vi "Set_Driver.vi"(8 "error in (no error)":errorcluster caption="错误输入（无错误）", 10 "Driver":string[](array[string]), 11 "文件路径 ：":path) -> (0 "error out":errorcluster, 3 "dup path":path)   [LabVIEW 2018]
uses:
  <vilib>/Utility/config.llb/Write Key (String).vi
  <vilib>/Utility/config.llb/NI_LVConfig.lvlib
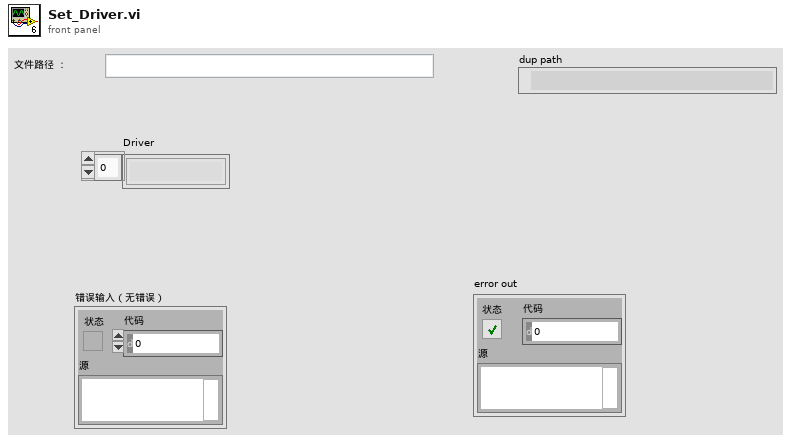
[diagram p1: front panel]
types:
  T1 = enum16{"open", "replace", "create", "open or create", "replace or create", "replace or create with confirmation"}
  T2 = typedef "NI_LVConfig.lvlib/Config Data RefNum.ctl" = refnum<k1>
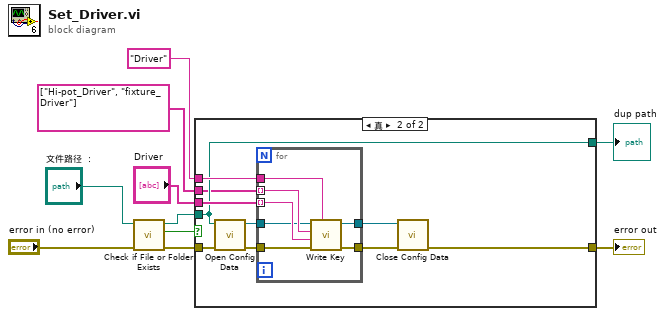
[diagram p0: block diagram]
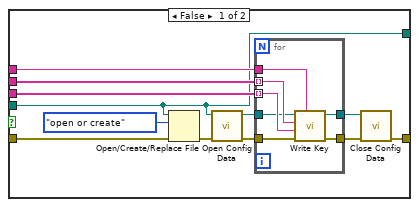
[diagram p2: hidden frame]
diagram:
  n1 = call <vilib>:"Check if File or Folder Exists.vi"("error in (no error)"="error in (no error)", "path"="文件路径 ：") -> ("error out"=w7:errorcluster, "file or folder exists?"=w9:bool, "dup path"=w8:path)  [unwired: 7 in]
  n2 = case shown="真" w9 {
    tunnel: w8 -> [w12 w33]
    tunnel: w7 -> [w14 w39]
    tunnel: "Driver" -> [w13 w38]
    tunnel: [w11 w37] -> w6
    tunnel: "Driver" -> [w18 w36]
    tunnel: [w12 w33] -> w10
    tunnel: string[] ["Hi-pot_Driver", "fixture_Driver"] -> [w17 w31]
    frame False {
      n3 = Open/Create/Replace File(file path (use dialog)=w12, error in=w14, operation (0:open)=T1."open or create" ("操作(0:open)")) -> (error out=w15:errorcluster)  [unwired: 3 in, 2 out]
      n4 = call <vilib>:"Open Config Data.vi"("error in (no error)"=w15, "configuration file path"=w12) -> ("error out"=w16:errorcluster, "refnum"=w19:T2)  [unwired: 7 in, 1 out]
      n5 = for {
        tunnel: w19 -> [w26]
        tunnel: w17 -> [w29] mode=indexing
        tunnel: w13 -> [w25]
        tunnel: w18 -> [w28] mode=indexing
        tunnel: [w27] -> w21
        tunnel: [w24] -> w20
        tunnel: w16 -> [w23]
        n6 = call-poly <vilib>:"Write Key.vi"("section"=w25, "error in (no error)"=w23, "value"=w28, "key"=w29, "refnum"=w26) -> ("error out"=w24:errorcluster, "refnum out"=w27:T2)  [unwired: 4 in, 1 out]
      }
      n7 = call <vilib>:"Close Config Data.vi"("error in (no error)"=w20, "refnum"=w21) -> ("error out"=w11:errorcluster)  [unwired: 8 in, 1 out]
    }
    frame True {
      n8 = call <vilib>:"Open Config Data.vi"("error in (no error)"=w39, "configuration file path"=w33) -> ("error out"=w32:errorcluster, "refnum"=w30:T2)  [unwired: 7 in, 1 out]
      n9 = for {
        tunnel: w30 -> [w43]
        tunnel: w31 -> [w46] mode=indexing
        tunnel: w38 -> [w42]
        tunnel: w36 -> [w45] mode=indexing
        tunnel: [w44] -> w35
        tunnel: [w41] -> w34
        tunnel: w32 -> [w40]
        n10 = call-poly <vilib>:"Write Key.vi"("section"=w42, "error in (no error)"=w40, "value"=w45, "key"=w46, "refnum"=w43) -> ("error out"=w41:errorcluster, "refnum out"=w44:T2)  [unwired: 4 in, 1 out]
      }
      n11 = call <vilib>:"Close Config Data.vi"("error in (no error)"=w34, "refnum"=w35) -> ("error out"=w37:errorcluster)  [unwired: 8 in, 1 out]
    }
  }
  "error out" <- w6
  "dup path" <- w10
